vi "solar_app Window.vi"(7 "Action (Set)":enum16{"Set", "Reset", "Clear"}(ring), 8 "error in (no error)":errorcluster, 9 "Target":string, 10 "VI Refnum":refnum<vi>, 11 "Config Path (*.ini)":path) -> (0 "error out":errorcluster)   [LabVIEW 2018]
doc: "This sets, resets or clears an unpinned target window position on the display monitor from the temporary configuration file."
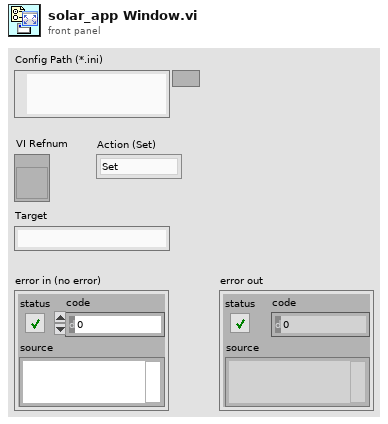
[diagram p1: front panel]
types:
  T1 = typedef "LVRectTypeDef.ctl" = cluster{"Left":i16, "Top":i16, "Right":i16, "Bottom":i16}
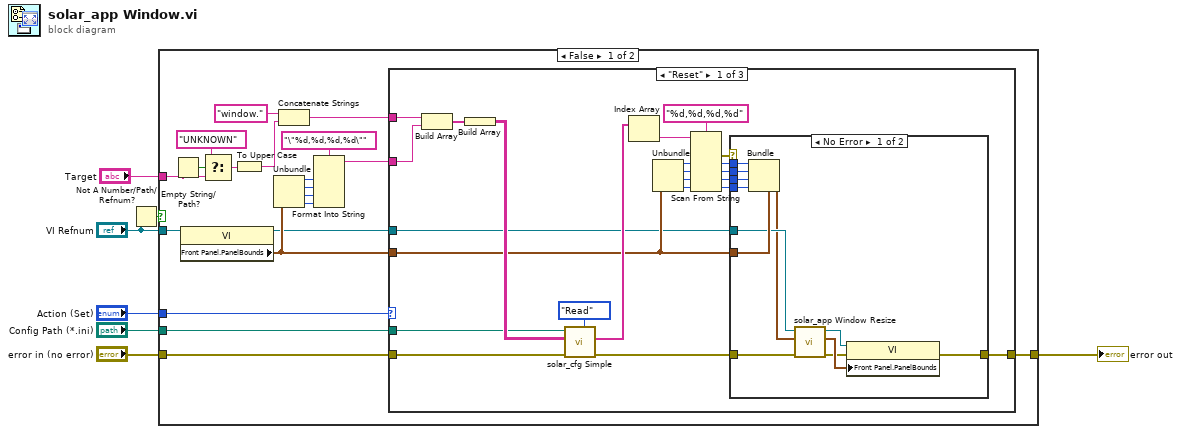
[diagram p0: block diagram]
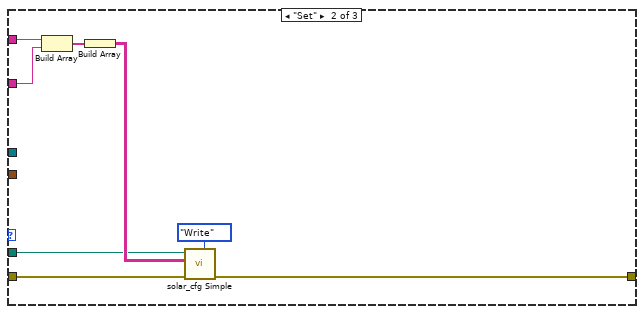
[diagram p3: hidden frame]
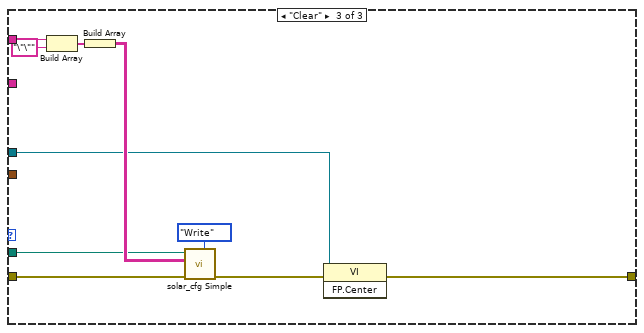
[diagram p4: hidden frame]
diagram:
  n1 = Not A Number/Path/Refnum?(number/path/refnum="VI Refnum") -> (NaN/Path/Refnum?=w3:bool)
  n2 = case shown="False" w3 {
    tunnel: "error in (no error)" -> [w16 w82]
    tunnel: "Config Path (*.ini)" -> [w15 _]
    tunnel: [w14 w82] -> w5
    tunnel: "Action (Set)" -> [w11 _]
    tunnel: "VI Refnum" -> [w8 _]
    tunnel: "Target" -> [w9 _]
    frame False {
      n3 = Empty String/Path?(string/path=w9) -> (empty?=w19:bool)
      n4 = property class="VI"(reference=w8) -> (reference out=w12:refnum<vi>, "Front Panel.PanelBounds"=w13:T1)  [unwired: 1 in, 1 out]
      n5 = Select(t="UNKNOWN", s=w19, f=w9) -> (s? t:f=w17:string)
      n6 = To Upper Case(1:w17) -> (0:w10:string)
      n7 = Unbundle(w13) -> ("Left"=w25:i16, "Top"=w24:i16, "Right"=w23:i16, "Bottom"=w22:i16)
      n8 = Concatenate Strings("window." ("String"), w10) -> (w26:string)
      n9 = Format Into String(format string="\"%d,%d,%d,%d\"", w25, w24, w23, w22) -> (resulting string=w20:string)  [unwired: 2 in, 1 out]
      n10 = case shown="\"Reset\"" w11 {
        tunnel: w26 -> [w49 w70 w80]
        tunnel: w20 -> [w48 w69 _]
        tunnel: w16 -> [w45 w66 w77]
        tunnel: w15 -> [w44 w65 w76]
        tunnel: [w39 w64 w73] -> w14
        tunnel: w13 -> [w30 _ _]
        tunnel: w12 -> [w29 _ w72]
        frame "Reset" {
          n11 = Build Array(w49, w48) -> (w47:string[])
          n12 = Build Array(w47) -> (w46:string[][])
          n13 = call "solar_cfg Simple.vi"("Action (Read)"=enum8{"Read", "Write"}."Read", "error in (no error)"=w45, "Key,Value,Comment"=w46, "Config Path (*.ini)"=w44) -> ("error out"=w40:errorcluster, "Values"=w43:string[])  [unwired: 4 in, 2 out]
          n14 = Index Array(array=w43) -> (element=w42:string)  [unwired: 1 in]
          n15 = Unbundle(w30) -> ("Left"=w34:i16, "Top"=w33:i16, "Right"=w32:i16, "Bottom"=w31:i16)
          n16 = Scan From String(format string="%d,%d,%d,%d", input string=w42, default 1=w34, default 2=w33, default 3=w32, default 4=w31) -> (error out=w28:errorcluster, output 1=w38:i16, output 2=w37:i16, output 3=w36:i16, output 4=w35:i16)  [unwired: 2 in, 2 out]
          n17 = case shown="No Error" w28 {
            tunnel: w40 -> [w62 w63]
            tunnel: [w51 w63] -> w39
            tunnel: w38 -> [w61 _]
            tunnel: w37 -> [w60 _]
            tunnel: w36 -> [w59 _]
            tunnel: w35 -> [w58 _]
            tunnel: w30 -> [w57 _]
            tunnel: w29 -> [w56 _]
            frame No Error {
              n18 = Bundle(cluster=w57, "Left"=w61, "Top"=w60, "Right"=w59, "Bottom"=w58) -> (w55:T1)
              n19 = call "solar_app Window Resize.vi"("error in (no error)"=w62, "New FP.WinBounds"=w55, "VI Refnum"=w56) -> ("error out"=w52:errorcluster, "Resolved FP.WinBounds"=w53:T1, "dup VI Refnum"=w54:refnum<vi>)  [unwired: 6 in]
              n20 = property class="VI"(reference=w54, error in=w52, "Front Panel.PanelBounds"=w53) -> (error out=w51:errorcluster)  [unwired: 1 out]
            }
            frame Error {
            }
          }
        }
        frame "Set" {
          n21 = Build Array(w70, w69) -> (w68:string[])
          n22 = Build Array(w68) -> (w67:string[][])
          n23 = call "solar_cfg Simple.vi"("Action (Read)"=enum8{"Read", "Write"}."Write", "error in (no error)"=w66, "Key,Value,Comment"=w67, "Config Path (*.ini)"=w65) -> ("error out"=w64:errorcluster)  [unwired: 4 in, 3 out]
        }
        frame "Clear" {
          n24 = Build Array(w80, "\"\"" ("element")) -> (w79:string[])
          n25 = Build Array(w79) -> (w78:string[][])
          n26 = call "solar_cfg Simple.vi"("Action (Read)"=enum8{"Read", "Write"}."Write", "error in (no error)"=w77, "Key,Value,Comment"=w78, "Config Path (*.ini)"=w76) -> ("error out"=w75:errorcluster)  [unwired: 4 in, 3 out]
          n27 = invoke class="VI" method="FP.Center"(reference=w72, error in=w75) -> (error out=w73:errorcluster)  [unwired: 1 in, 2 out]
        }
      }
    }
    frame True {
    }
  }
  "error out" <- w5
